vi "nelder_make_initial_simplex.vi"(6 "error in (no error)":errorcluster, 7 "settling time":u32, 8 "initial simplex":T1, 9 "References":T3) -> (0 "error out":errorcluster, 3 "output simplex":sgl[][](array[numeric]))   [LabVIEW 2018]
uses:
  C:/Program Files/National Instruments/LabVIEW 2018/instr.lib/IDS/ueye.NET/uEyeDotNet.dll
  <userlib>/PDamp/PDref.ctl
  <userlib>/PDamp/channel.ctl
  cb2c0b56-3610-43b6-a560-85e423fae6a7.vi
  <vilib>/Array/Sort 2D Array - Pop Stack.vi
  <vilib>/Array/Sort 2D Array - Push Stack.vi
  cb2c0b56-3610-43b6-a560-85e423fae6a7.vi/fc8878de-6f79-43c3-83a5-482868420899.vi
  cb2c0b56-3610-43b6-a560-85e423fae6a7.vi/4f1a352b-3e21-4927-85f9-d1111eff9dd0.vi
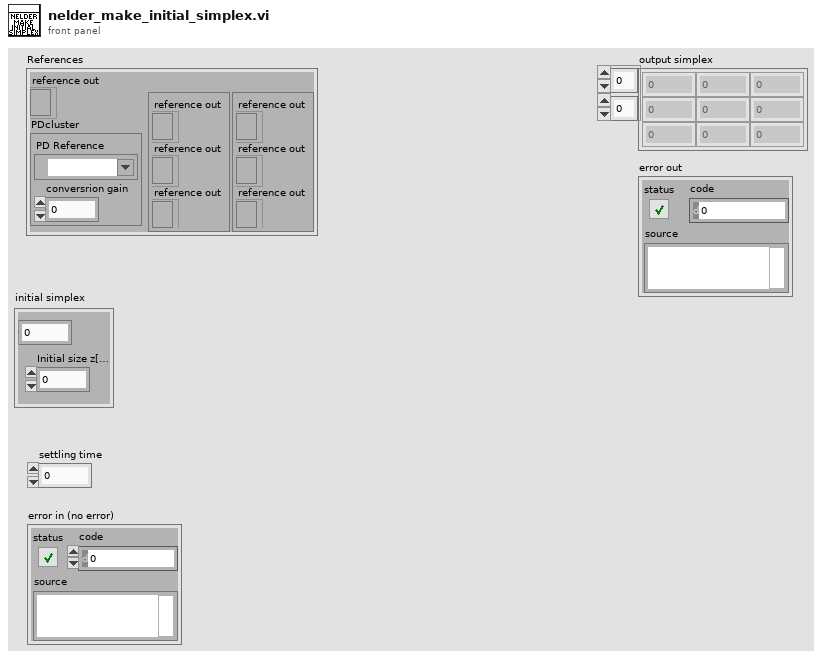
[diagram p1: front panel]
types:
  T1 = cluster{"Initial size y[µm]":sgl, "Initial size z[µm]":sgl}
  T2 = typedef "PDref.ctl" = cluster{"PD Reference":refnum<visa-resource-name>, "conversrion gain":dbl}
  T3 = cluster{"reference out":refnum<k24>, "PDcluster":T2, cluster{"reference out":refnum<k7>, "reference out":refnum<k7>, "reference out":refnum<k7>}, cluster{"reference out":refnum<k7>, "reference out":refnum<k7>, "reference out":refnum<k7>}}
  T4 = cluster{"reference out":refnum<k7>, "reference out":refnum<k7>, "reference out":refnum<k7>}
  T5 = typedef "channel.ctl" = enum16{"ch1", "ch2", "ch3", "ch4"}
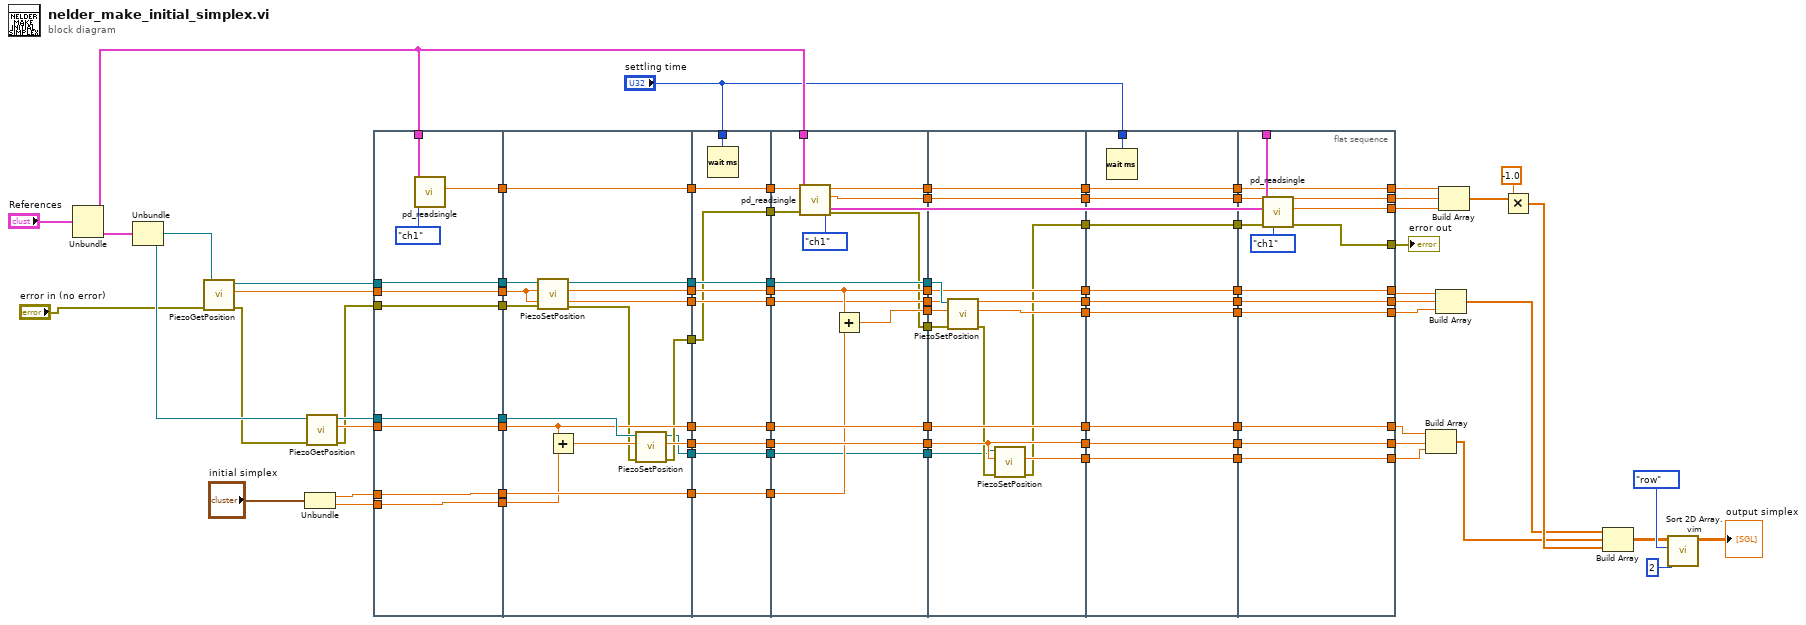
[diagram p0: block diagram]
diagram:
  n1 = Unbundle("References") -> ("PDcluster"=w77:T2, w78:T4)  [unwired: 2 out]
  n2 = Unbundle(w78) -> ("reference out"=w89:refnum<k7>, "reference out"=w88:refnum<k7>)  [unwired: 1 out]
  n3 = call <userlib>:"PiezoGetPosition.vi"("error in (no error)"="error in (no error)", "reference"=w89) -> ("error out"=w29:errorcluster, "Position"=w75:sgl, "reference out"=w60:refnum<k7>)  [unwired: 3 in]
  n4 = Unbundle("initial simplex") -> ("Initial size y[µm]"=w6:sgl, "Initial size z[µm]"=w4:sgl)
  n5 = call <userlib>:"PiezoGetPosition.vi"("error in (no error)"=w29, "reference"=w88) -> ("error out"=w28:errorcluster, "Position"=w56:sgl, "reference out"=w59:refnum<k7>)  [unwired: 3 in]
  n6 = flat-sequence {
    tunnel: w75 -> [w99]
    tunnel: [w99] -> w87
    tunnel: w77 -> [w98]
    tunnel: [w96] -> w70
    tunnel: w60 -> [w95]
    tunnel: [w95] -> w61
    tunnel: w59 -> [w94]
    tunnel: [w94] -> w58
    tunnel: [w93] -> w57
    tunnel: w56 -> [w93]
    tunnel: w28 -> [w92]
    tunnel: [w92] -> w27
    tunnel: [w91] -> w7
    tunnel: w6 -> [w91]
    tunnel: [w90] -> w5
    tunnel: w4 -> [w90]
    tunnel: w87 -> [w108]
    tunnel: [w112] -> w84
    tunnel: [w111] -> w71
    tunnel: w70 -> [w111]
    tunnel: w61 -> [w110]
    tunnel: w58 -> [w109]
    tunnel: w57 -> [w107]
    tunnel: [w108] -> w55
    tunnel: [w108] -> w48
    tunnel: [w107] -> w42
    tunnel: [w106] -> w41
    tunnel: w27 -> [w105]
    tunnel: [w103] -> w26
    tunnel: [w102] -> w8
    tunnel: w7 -> [w102]
    tunnel: w5 -> [w101]
    tunnel: [w100] -> w3
    tunnel: [w122] -> w85
    tunnel: w84 -> [w122]
    tunnel: "settling time" -> [w121]
    tunnel: [w120] -> w72
    tunnel: w71 -> [w120]
    tunnel: w55 -> [w119]
    tunnel: [w119] -> w54
    tunnel: w48 -> [w118]
    tunnel: [w118] -> w47
    tunnel: w42 -> [w117]
    tunnel: w41 -> [w116]
    tunnel: [w117] -> w37
    tunnel: [w116] -> w35
    tunnel: w26 -> [w115]
    tunnel: [w115] -> w25
    tunnel: [w114] -> w9
    tunnel: w8 -> [w114]
    tunnel: w3 -> [w113]
    tunnel: [w113] -> w2
    tunnel: w77 -> [w135]
    tunnel: [w134] -> w86
    tunnel: w85 -> [w134]
    tunnel: [w133] -> w73
    tunnel: w72 -> [w133]
    tunnel: [w132] -> w66
    tunnel: w54 -> [w130]
    tunnel: [w131] -> w53
    tunnel: [w130] -> w51
    tunnel: w47 -> [w129]
    tunnel: [w129] -> w44
    tunnel: [w128] -> w38
    tunnel: w37 -> [w128]
    tunnel: [w127] -> w36
    tunnel: w35 -> [w127]
    tunnel: w25 -> [w126]
    tunnel: [w125] -> w24
    tunnel: w9 -> [w124]
    tunnel: w2 -> [w123]
    tunnel: [w123] -> w1
    tunnel: w86 -> [w148]
    tunnel: [w147] -> w74
    tunnel: w73 -> [w147]
    tunnel: [w146] -> w67
    tunnel: w66 -> [w146]
    tunnel: w53 -> [w145]
    tunnel: [w145] -> w52
    tunnel: w51 -> [w144]
    tunnel: [w144] -> w50
    tunnel: [w143] -> w45
    tunnel: w44 -> [w143]
    tunnel: [w142] -> w39
    tunnel: w38 -> [w142]
    tunnel: w36 -> [w141]
    tunnel: [w141] -> w34
    tunnel: [w141] -> w33
    tunnel: w24 -> [w140]
    tunnel: [w138] -> w22
    tunnel: w1 -> [w137]
    tunnel: "settling time" -> [w158]
    tunnel: w74 -> [w157]
    tunnel: [w157] -> w69
    tunnel: [w156] -> w68
    tunnel: w67 -> [w156]
    tunnel: w52 -> [w153]
    tunnel: w50 -> [w155]
    tunnel: [w155] -> w49
    tunnel: [w154] -> w46
    tunnel: w45 -> [w154]
    tunnel: [w153] -> w43
    tunnel: [w152] -> w40
    tunnel: w39 -> [w152]
    tunnel: w34 -> [w151]
    tunnel: w33 -> [w150]
    tunnel: [w151] -> w32
    tunnel: [w150] -> w31
    tunnel: [w149] -> w23
    tunnel: w22 -> [w149]
    tunnel: w77 -> [w171]
    tunnel: [w169] -> w63
    tunnel: w69 -> [w169]
    tunnel: w68 -> [w168]
    tunnel: [w168] -> w62
    tunnel: [w167] -> w65
    tunnel: w49 -> [w166]
    tunnel: [w166] -> w19
    tunnel: [w165] -> w18
    tunnel: w46 -> [w165]
    tunnel: [w164] -> w17
    tunnel: w43 -> [w164]
    tunnel: [w163] -> w14
    tunnel: w40 -> [w163]
    tunnel: w32 -> [w161]
    tunnel: [w162] -> w13
    tunnel: w31 -> [w162]
    tunnel: [w161] -> w15
    tunnel: w23 -> [w160]
    tunnel: [w159] -> w21
    frame #0 {
      n7 = call <userlib>:"pd_readsingle.vi"("PDcluster in"=w98, "channel"=channel."ch1") -> ("photocurrent"=w96:dbl)  [unwired: 6 in, 2 out]
    }
    frame #1 {
      n8 = call <userlib>:"PiezoSetPosition.vi"("error in (no error)"=w105, "pos in"=w108, "reference"=w110) -> ("error out"=w104:errorcluster, "reference out"=w112:refnum<k7>)  [unwired: 3 in]
      n9 = Add(x=w107, y=w101) -> (x+y=w106:sgl)
      n10 = call <userlib>:"PiezoSetPosition.vi"("error in (no error)"=w104, "pos in"=w106, "reference"=w109) -> ("error out"=w103:errorcluster, "reference out"=w100:refnum<k7>)  [unwired: 3 in]
    }
    frame #2 {
      n11 = Wait (ms)(milliseconds to wait=w121) -> ()  [unwired: 1 out]
    }
    frame #3 {
      n12 = call <userlib>:"pd_readsingle.vi"("PDcluster in"=w135, "channel"=channel."ch1", "error in (no error)"=w126) -> ("photocurrent"=w132:dbl, "error out"=w125:errorcluster)  [unwired: 5 in, 1 out]
      n13 = Add(x=w130, y=w124) -> (x+y=w131:sgl)
    }
    frame #4 {
      n14 = call <userlib>:"PiezoSetPosition.vi"("error in (no error)"=w140, "pos in"=w145, "reference"=w148) -> ("error out"=w139:errorcluster)  [unwired: 3 in, 1 out]
      n15 = call <userlib>:"PiezoSetPosition.vi"("error in (no error)"=w139, "pos in"=w141, "reference"=w137) -> ("error out"=w138:errorcluster)  [unwired: 3 in, 1 out]
    }
    frame #5 {
      n16 = Wait (ms)(milliseconds to wait=w158) -> ()  [unwired: 1 out]
    }
    frame #6 {
      n17 = call <userlib>:"pd_readsingle.vi"("PDcluster in"=w171, "channel"=channel."ch1", "error in (no error)"=w160) -> ("photocurrent"=w167:dbl, "error out"=w159:errorcluster)  [unwired: 5 in, 1 out]
    }
  }
  n18 = Build Array(w14, w15, w13) -> (w12:sgl[])
  n19 = Build Array(w19, w18, w17) -> (w16:sgl[])
  n20 = Build Array(w63, w62, w65) -> (w80:dbl[])
  n21 = Multiply(x=w80, y=-1.0 ("output")) -> (x*y=w20:dbl[])
  n22 = Build Array(w16, w12, w20) -> (w11:dbl[][])
  n23 = call "Sort 2D Array.vim"("index"=2, "dimension to index (column)"=enum16{"column", "row"}."row", "2D array"=w11) -> ("sorted 2D array"=→"output simplex":dbl[][])  [unwired: 7 in, 1 out]
  "error out" <- w21
